vi "Global - Done.vi"() -> ()   [LabVIEW 2019]
panel:
  in  "Done":bool[](array[boolean])=[FALSE, FALSE, FALSE, FALSE, FALSE, FALSE, FALSE, FALSE, FALSE, FALSE]
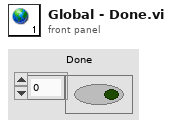
[diagram p1: front panel]
diagram:
